vi "DMAC U8 to DMAC String.vi"(5 "DestinationMACAddress":u8[](array[numeric])=[3, 0, 94, 160, 3, 233] format="%02x") -> (2 "DMAC String":string)   [LabVIEW 2021, in "Networking_CIF_U.lvlib"]
uses:
  Networking_CIF_U.lvlib
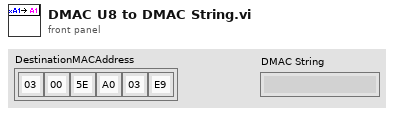
[diagram p1: front panel]
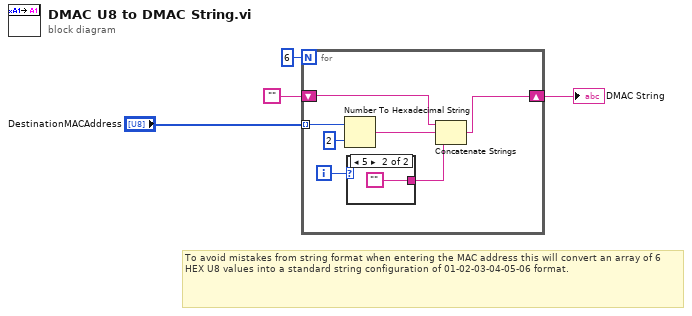
[diagram p0: block diagram]
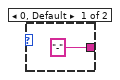
[diagram p2: hidden frame]
diagram:
  # "To avoid mistakes from string format when entering the MAC address this will convert an array of 6 HEX U8 values into a standard string configuration of 01-02-03-04-05-06 format."
  n1 = for {
    N: 6 -> [_]
    tunnel: "DestinationMACAddress" -> [w11] mode=indexing
    shift-right: [w6] -> w1
    shift-left: "" -> [w9]
    i -> [w5]
    n2 = Number To Hexadecimal String(1:i16 2 ("width (-)"), 2:w11) -> (0:w8:string)
    n3 = case shown="5" w5 {
      tunnel: ["-" ""] -> w7
      frame 0, Default {
      }
      frame 5 {
      }
    }
    n4 = Concatenate Strings(w9, w8, w7) -> (w6:string)
  }
  "DMAC String" <- w1
